vi "Teleop.vi"(10 "Match Info":T1={"Autonomous Elapsed Seconds"=0.0, "TeleOp Elapsed Seconds"=0.0, "Disabled Elapsed Seconds"=0.0, "Visited Autonomous"=FALSE, "Visited TeleOp"=FALSE, "Visited Disabled"=FALSE, "Autonomous Settings"={"Autonomous Style"=enum."Independent", "VI Refnum"=refnum}}, 11 "Call Context":T2) -> ()   [LabVIEW 2015]
doc: "This VI is called for each TeleOp packet received from the DS where the robot is not disabled. It is often used to read from the joysticks and update I/O or to update setpoints for timed control loops. It should complete and return within 20 milliseconds or it may miss DS packets."
uses:
  <vilib>/Rock Robotics/WPI/DriverStation/WPI_DriverStationDerivedRobotMode.ctl
  <vilib>/Rock Robotics/WPI/DriverStation/WPI_DriverStationMatch Info.ctl
  <vilib>/Rock Robotics/Network Tables/NT Read Boolean.vi
  <vilib>/Rock Robotics/Network Tables/NT Read Number.vi
  <vilib>/Rock Robotics/WPI/Utilities/WPI_GetSetVariantRefNum.vi
  <vilib>/Rock Robotics/Network Tables/NT Write Boolean Array.vi
  <vilib>/Rock Robotics/Network Tables/NT Write Numeric Array.vi
  <vilib>/Rock Robotics/Network Tables/NT Write Boolean.vi
  <vilib>/Rock Robotics/WPI/Solenoid/Deprecated/WPI_SolenoidSetBool.vi
  Sensors.vi
  Robot Global Data.vi
panel:
  in  "t":dbl=0.9
  in  "y":dbl=22500.0 format="%#_13g"
  out "Done":bool
  out "Drive Over":bool
  out "Start Climbing":bool
  out "Slow Turning":bool
  in  "Joystick Toning Factor":dbl=0.8 format="%#_13g"
  out "Release Climber Head":bool
  out "Release Climbing Solenoid":bool
  out "Break":bool
  out "Roller Open":bool
  out "Correct Wire":bool
  out "Alignment line shot":bool
  out "Low Goal":bool
  out "Lock Release":bool
  out "Auto Vision Tracking":bool
  out "High Goal shoot":bool
  out "High Goal prep":bool
  out "Intake Start":bool
  out "Sample Slider 0":dbl(slide) scale=0.0..5.0
  out "Sample Boolean 1":bool
  out "Sample Boolean 0":bool
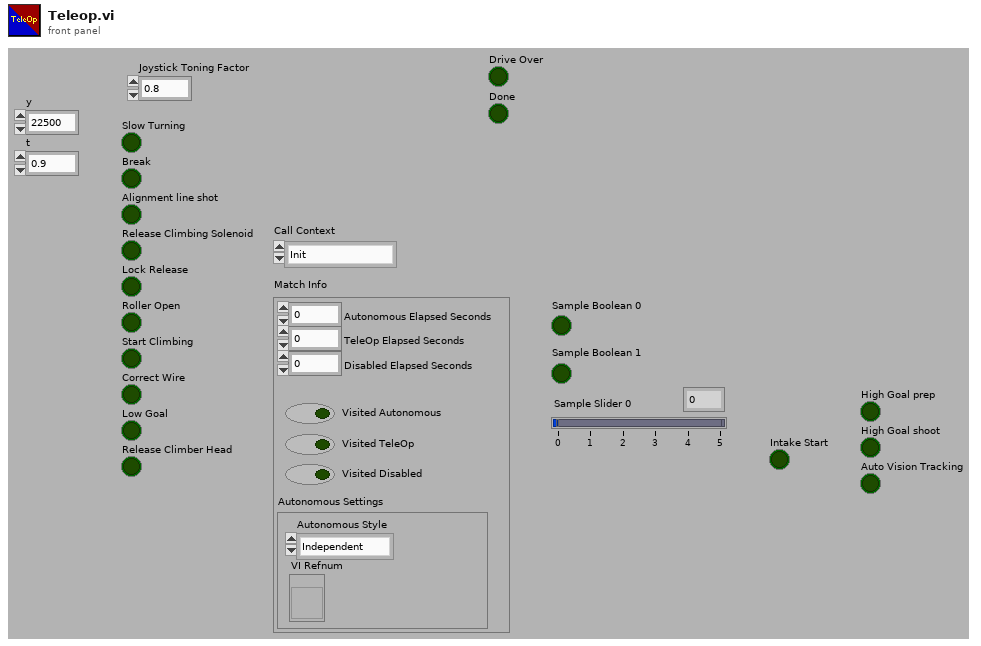
[diagram p1: front panel]
types:
  T1 = typedef "WPI_DriverStationMatch Info.ctl" = cluster{"Autonomous Elapsed Seconds":dbl, "TeleOp Elapsed Seconds":dbl, "Disabled Elapsed Seconds":dbl, "Visited Autonomous":bool, "Visited TeleOp":bool, "Visited Disabled":bool, "Autonomous Settings":cluster{"Autonomous Style":enum16{"Iterative", "Independent"}, "VI Refnum":refnum<vi>}}
  T2 = typedef "WPI_DriverStationDerivedRobotMode.ctl" = enum16{"Init", "Execute", "Stop"}
  T3 = typedef "WPI_JoystickDevRef.ctl" = cluster{"Device":T4}
  T4 = typedef "WPI_JoystickDeviceEnum.ctl" = enum16{"USB 0", "USB 1", "USB 2", "USB 3", "USB 4", "USB 5"}
  T5 = typedef "WPI_DigitalInputDevRef.ctl" = cluster{"DevStatus":errorcluster, "DIO Channel":T6}
  T6 = typedef "FPGA_DIOChannel.ctl" = enum8{"DIO 0", "DIO 1", "DIO 2", "DIO 3", "DIO 4", "DIO 5", "DIO 6", "DIO 7", "DIO 8", "DIO 9", "DIO MXP 0", "DIO MXP 1", "DIO MXP 2", "DIO MXP 3", "DIO MXP 4", "DIO MXP 5", "DIO MXP 6", "DIO MXP 7", "DIO MXP 8", "DIO MXP 9", "DIO MXP 10", "DIO MXP 11", "DIO MXP 12", "DIO MXP 13", "DIO MXP 14", "DIO MXP 15", "Invalid"}
  T7 = typedef "WPI_MotorControlDeviceRef.ctl" = cluster{"DeviceStatus":errorcluster, "Type":T8, "PWM":cluster{"PWM Channel":T9, "DeadBand":T10}, "CAN":cluster{"Device Number":u8, "Control Mode":T11, "Semaphore":T12, "Max Vout":dbl, "TalonSRX Control Mode":T13}, "Invert":bool}
  T8 = typedef "WPI_MotorControlType.ctl" = enum16{"PWM", "CAN", "CANTalonSRX"}
  T9 = typedef "FPGA_DIOPWMChannel.ctl" = enum8{"PWM 0", "PWM 1", "PWM 2", "PWM 3", "PWM 4", "PWM 5", "PWM 6", "PWM 7", "PWM 8", "PWM 9", "PWM MXP 0", "PWM MXP 1", "PWM MXP 2", "PWM MXP 3", "PWM MXP 4", "PWM MXP 5", "PWM MXP 6", "PWM MXP 7", "PWM MXP 8", "PWM MXP 9", "Invalid"}
  T10 = typedef "WPI_PWMDeadband.ctl" = cluster{"Name":string, "maxPositivePwm":i32, "minPositivePwm":i32, "centerPwm":i32, "maxNegativePwm":i32, "minNegativePwm":i32, "angularRange":u16}
  T11 = typedef "WPI_CANJaguar_ControlMode.ctl" = enum8{"Percent VBus", "Current", "Speed", "Position", "Voltage"}
  T12 = typedef "Semaphore RefNum" = refnum<k1>
  T13 = typedef "WPI_CANTalonSRX_APIControlMode.ctl" = enum8{"Percent VBus", "Speed", "Position", "Slave", "Unchanged / Invalid", "Voltage Compensation", "Current", "Motion Profile"}
  T14 = typedef "WPI_RobotDriveDevRef.ctl" = cluster{"DevStatus":errorcluster, "Motors[]":T7[], "Square Inputs":bool, "Max Output":dbl}
  T15 = typedef "WPI_SolenoidDevRef.ctl" = cluster{"DevStatus":errorcluster, "Pneumatics Control Module":u8, "Forward Solenoid Channel":T16, "Reverse Solenoid Channel":T16}
  T16 = typedef "WPI_SolenoidChannel.ctl" = enum8{"Solenoid 0", "Solenoid 1", "Solenoid 2", "Solenoid 3", "Solenoid 4", "Solenoid 5", "Solenoid 6", "Solenoid 7", "Invalid"}
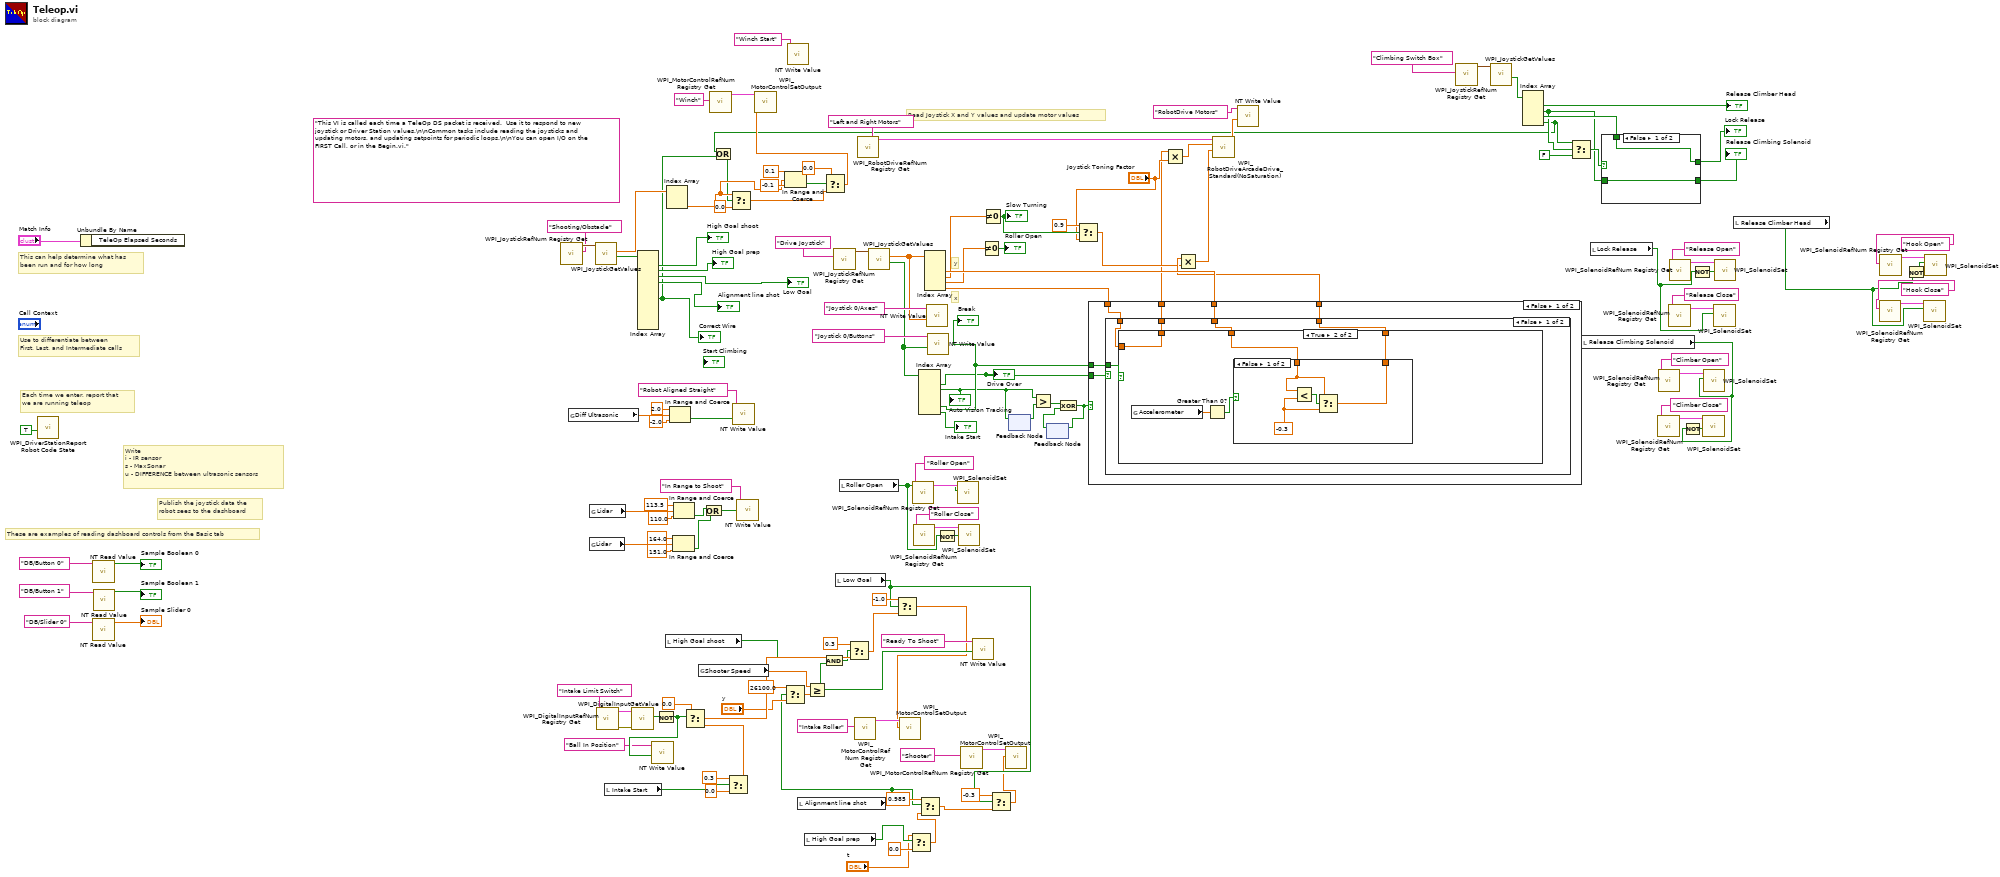
[diagram p0: block diagram]
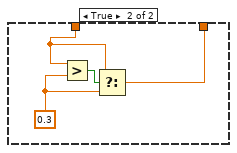
[diagram p3: hidden frame]
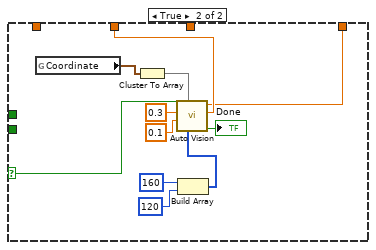
[diagram p5: hidden frame]
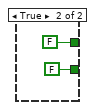
[diagram p6: hidden frame]
diagram:
  (unwired) "This VI is called each time a TeleOp DS packet is received.  Use it to respond to new joystick or Driver Station values.\n\nCommon tasks include reading the joysticks and updating motors, and updating setpoints for periodic loops.\n\nYou can open I/O on the FIRST Call, or in the Begin.vi."
  # "x"
  # "y"
  # "Read Joystick X and Y values and update motor values"
  # "Write\ni - IR sensor\ns - MaxSonar\nu - DIFFERENCE between ultrasonic sensors"
  # "These are examples of reading dashboard controls from the Basic tab"
  # "Publish the joystick data the\nrobot sees to the dashboard"
  # "Each time we enter, report that\nwe are running teleop"
  # "Use to differentiate between\nFirst, Last, and Intermediate calls"
  # "This can help determine what has\nbeen run and for how long"
  n1 = call <vilib>:"WPI_DriverStationReport Robot Code State.vi"("TeleOp"=TRUE ("Autonomous")) -> ()  [unwired: 10 in, 1 out]
  n2 = Unbundle By Name("Match Info") -> ()  [unwired: 1 out]
  n3 = call-poly <vilib>:"NT Read Value.vi"("Name"="DB/Button 0" ("refnum name")) -> ("Boolean"=→"Sample Boolean 0":bool)  [unwired: 9 in, 1 out]
  n4 = call-poly <vilib>:"NT Read Value.vi"("Name"="DB/Slider 0" ("refnum name")) -> ("Numeric"=→"Sample Slider 0":dbl)  [unwired: 9 in, 1 out]
  n5 = call-poly <vilib>:"NT Read Value.vi"("Name"="DB/Button 1" ("refnum name")) -> ("Boolean"=→"Sample Boolean 1":bool)  [unwired: 9 in, 1 out]
  n6 = call <vilib>:"WPI_JoystickRefNum Registry Get.vi"("refnum name"="Shooting/Obstacle") -> ("JoystickDevRef"=w122:T3)  [unwired: 1 in, 9 out]
  n7 = global read "Sensors.vi" "Diff Ultrasonic"() -> (w51:dbl)
  n8 = global read "Sensors.vi" "Lidar"() -> (w42:dbl)
  n9 = global read "Sensors.vi" "Lidar"() -> (w43:dbl)
  n10 = call <vilib>:"WPI_JoystickGetValues.vi"("JoystickDevRef"=w122) -> ("Buttons"=w120:bool[], "Axes"=w118:dbl[])  [unwired: 6 in, 3 out]
  n11 = call <vilib>:"WPI_DigitalInputRefNum Registry Get.vi"("refnum name"="Intake Limit Switch") -> ("error out"=w105:errorcluster, "DigitalInputDevRef"=w106:T5)  [unwired: 9 in]
  n12 = local read "Intake Start"() -> (w103:bool)
  n13 = call <vilib>:"WPI_DigitalInputGetValue.vi"("error in (no error)"=w105, "DigitalInputDevRef"=w106) -> ("Value"=w108:bool)  [unwired: 7 in, 2 out]
  n14 = Index Array(array=w120) -> (element #1=→"High Goal shoot":bool, element #2=→"High Goal prep":bool, element #3=→"Low Goal":bool, element #4=→"Alignment line shot":bool, element #7=w5:bool)  [unwired: 12 in, 7 out]
  "Correct Wire" <- w5
  n15 = Not(x=w108) -> (.not. x?=w58:bool)
  n16 = call-poly <vilib>:"NT Write Value.vi"("Boolean"=w58, "Name"="Ball In Position") -> ()  [unwired: 9 in, 1 out]
  n17 = local read "High Goal shoot"() -> (w95:bool)
  n18 = Index Array(array=w118) -> (element #2=w60:dbl)  [unwired: 2 in, 1 out]
  n19 = In Range and Coerce(upper limit=2.0, x=w51, lower limit=-2.0) -> (In Range?=w48:bool)  [unwired: 1 out]
  n20 = In Range and Coerce(upper limit=164.0, x=w42, lower limit=151.0) -> (In Range?=w38:bool)  [unwired: 1 out]
  n21 = In Range and Coerce(upper limit=113.5, x=w43, lower limit=110.0) -> (In Range?=w39:bool)  [unwired: 1 out]
  n22 = global read "Sensors.vi" "Shooter Speed"() -> (w1:dbl)
  n23 = Or(x=w39, y=w38) -> (x .or. y?=w37:bool)
  n24 = call <vilib>:"WPI_MotorControlRefNum Registry Get.vi"("refnum name"="Winch") -> ("MotorControlDevRef"=w80:T7)  [unwired: 9 in, 1 out]
  n25 = Select(t=0.3, s=w103, f=0.0) -> (s? t:f=w100:dbl)
  n26 = Select(t=0.0, s=w58, f=w100) -> (s? t:f=w99:dbl)
  n27 = call-poly <vilib>:"NT Write Value.vi"("Boolean"=w48, "Name"="Robot Aligned Straight") -> ()  [unwired: 9 in, 1 out]
  n28 = call-poly <vilib>:"NT Write Value.vi"("Boolean"=w37, "Name"="In Range to Shoot") -> ()  [unwired: 9 in, 1 out]
  n29 = In Range and Coerce(upper limit=0.1, x=w60, lower limit=-0.1) -> (In Range?=w76:bool)  [unwired: 1 out]
  n30 = call-poly <vilib>:"NT Write Value.vi"("Name"="Winch Start") -> ()  [unwired: 10 in, 1 out]
  n31 = local read "Alignment line shot"() -> (w29:bool)
  n32 = Select(t=26100.0, s=w29, f="y") -> (s? t:f=w30:dbl)
  n33 = local read "High Goal prep"() -> (w97:bool)
  n34 = Greater Or Equal?(x=w1, y=w30) -> (x >= y?=w55:bool)
  n35 = And(x=w95, y=w55) -> (x .and. y?=w94:bool)
  n36 = call <vilib>:"WPI_JoystickRefNum Registry Get.vi"("refnum name"="Drive Joystick") -> ("JoystickDevRef"=w128:T3)  [unwired: 1 in, 9 out]
  n37 = local read "Low Goal"() -> (w53:bool)
  n38 = local read "Roller Open"() -> (w109:bool)
  n39 = Select(t=0.3, s=w94, f=w99) -> (s? t:f=w111:dbl)
  n40 = call <vilib>:"WPI_MotorControlRefNum Registry Get.vi"("refnum name"="Intake Roller") -> ("MotorControlDevRef"=w132:T7)  [unwired: 9 in, 1 out]
  n41 = call <vilib>:"WPI_RobotDriveRefNum Registry Get.vi"("refnum name"="Left and Right Motors") -> ("RobotDriveDevRef"=w130:T14)  [unwired: 1 in, 9 out]
  n42 = call <vilib>:"WPI_JoystickGetValues.vi"("JoystickDevRef"=w128) -> ("Buttons"=w123:bool[], "Axes"=w119:dbl[])  [unwired: 6 in, 3 out]
  n43 = Select(t=-1.0, s=w53, f=w111) -> (s? t:f=w35:dbl)
  n44 = call <vilib>:"WPI_MotorControlSetOutput.vi"("Output"=w35, "MotorControlDevRef"=w132) -> ()  [unwired: 7 in, 3 out]
  n45 = Select(t="t", s=w97, f=0.0) -> (s? t:f=w28:dbl)
  n46 = call <vilib>:"WPI_SolenoidRefNum Registry Get.vi"("refnum name"="Roller Open") -> ("SolenoidDevRef"=w139:T15)  [unwired: 9 in, 1 out]
  n47 = call <vilib>:"WPI_SolenoidRefNum Registry Get.vi"("refnum name"="Roller Close") -> ("SolenoidDevRef"=w136:T15)  [unwired: 9 in, 1 out]
  n48 = Index Array(array=w123) -> (element #1=w36:bool, element #2=w12:bool, element #5=w92:bool, element #6=→"Intake Start":bool)  [unwired: 6 in, 2 out]
  "Auto Vision Tracking" <- w12
  "Break" <- w92
  "Drive Over" <- w36
  n49 = Select(t=0.985, s=w29, f=w28) -> (s? t:f=w32:dbl)
  n50 = Index Array(array=w119) -> (element #2=w93:dbl, element #3=w66:dbl, element #4=w69:dbl, element #5=w7:dbl)  [unwired: 5 in, 1 out]
  n51 = call-poly <vilib>:"NT Write Value.vi"("Numeric Array"=w119, "Name"="Joystick 0/Axes") -> ()  [unwired: 9 in, 1 out]
  n52 = call-poly <vilib>:"NT Write Value.vi"("Boolean Array"=w123, "Name"="Joystick 0/Buttons") -> ()  [unwired: 9 in, 1 out]
  n53 = Not(x=w109) -> (.not. x?=w135:bool)
  n54 = call-poly <vilib>:"WPI_SolenoidSet.vi"("Value"=w109, "SolenoidDevRef"=w139) -> ()  [unwired: 8 in, 2 out]
  n55 = call-poly <vilib>:"WPI_SolenoidSet.vi"("Value"=w135, "SolenoidDevRef"=w136) -> ()  [unwired: 8 in, 2 out]
  n56 = call <vilib>:"WPI_MotorControlRefNum Registry Get.vi"("refnum name"="Shooter") -> ("MotorControlDevRef"=w133:T7)  [unwired: 9 in, 1 out]
  n57 = call-poly <vilib>:"NT Write Value.vi"("Boolean"=w55, "Name"="Ready To Shoot") -> ()  [unwired: 9 in, 1 out]
  n58 = Not Equal To 0?(x=w69) -> (x != 0?=→"Roller Open":bool)
  n59 = Not Equal To 0?(x=w66) -> (x != 0?=w65:bool)
  "Slow Turning" <- w65
  n60 = Select(t=-0.3, s=w53, f=w32) -> (s? t:f=w34:dbl)
  n61 = call <vilib>:"WPI_MotorControlSetOutput.vi"("Output"=w34, "MotorControlDevRef"=w133) -> ()  [unwired: 7 in, 3 out]
  n62 = feedback-in #1(w12) -> ()
  n63 = feedback #1() -> (w13:bool)  [unwired: 1 in]
  n64 = Greater?(x=w12, y=w13) -> (0:w9:bool)
  n65 = feedback #2() -> (w10:bool)  [unwired: 1 in]
  n66 = Exclusive Or(1:w10, 2:w9) -> (0:w11:bool)
  n67 = feedback-in #2(w11) -> ()
  n68 = Select(t=0.9, s=w65, f="Joystick Toning Factor") -> (s? t:f=w62:dbl)
  n69 = case shown="False" w11 {
    selector: w11 -> [_ w182]
    tunnel: w93 -> [w154 _]
    tunnel: w92 -> [w153 _]
    tunnel: [w152 w177] -> w72
    tunnel: w36 -> [w151 _]
    tunnel: [w150 w178] -> w8
    tunnel: w7 -> [w149 _]
    frame False {
      n70 = case shown="False" w151 {
        tunnel: w154 -> [w159 w175]
        tunnel: w153 -> [w158 _]
        tunnel: [w157 w175] -> w152
        tunnel: [w156 w176] -> w150
        tunnel: w149 -> [w155 w176]
        frame False {
          n71 = case shown="True" w158 {
            tunnel: w159 -> [w161 w163]
            tunnel: [w161 w162] -> w157
            tunnel: [w160 w166] -> w156
            tunnel: w155 -> [w160 w166]
            frame False {
            }
            frame True {
              n72 = global read "Sensors.vi" "Accelerometer"() -> (w164:dbl)
              n73 = Greater Than 0?(x=w164) -> (x > 0?=w165:bool)
              n74 = case shown="False" w165 {
                tunnel: w163 -> [w168 w173]
                tunnel: [w167 w171] -> w162
                frame False {
                  w169 = -0.3
                  n75 = Less?(x=w168, y=w169) -> (x < y?=w170:bool)
                  n76 = Select(t=w168, s=w170, f=w169) -> (s? t:f=w167:dbl)
                }
                frame True {
                  w172 = 0.3
                  n77 = Greater?(x=w173, y=w172) -> (0:w174:bool)
                  n78 = Select(t=w173, s=w174, f=w172) -> (s? t:f=w171:dbl)
                }
              }
            }
          }
        }
        frame True {
        }
      }
    }
    frame True {
      n79 = global read "Robot Global Data.vi" "Coordinate"() -> (w185:cluster{"X":dbl, "Y":dbl})
      n80 = Cluster To Array(cluster=w185) -> (array=w183:dbl[])
      n81 = Build Array(160, 120) -> (w180:i32[])
      n82 = call "Auto Vision.vi"("Image Size"=w180, "Max Coordinate"=w183, "Rotational Velocity"=0.1, "Linear Velocity"=0.3, "Follow Colour ON"=w182) -> ("Done"=→"Done":bool, "Rotational Velocity_After"=w178:dbl, "Translational Velocity_After"=w177:dbl)  [unwired: 4 in]
    }
  }
  n83 = Multiply(x=w8, y="Joystick Toning Factor") -> (x*y=w73:dbl)
  n84 = Multiply(x=w72, y=w62) -> (x*y=w71:dbl)
  n85 = call <vilib>:"WPI_RobotDriveArcadeDrive_Standard(NoSaturation).vi"("Y axis value"=w71, "X axis value"=w73, "RobotDriveDevRef"=w130) -> ("Motor Values"=w125:dbl[])  [unwired: 1 in, 7 out]
  n86 = call-poly <vilib>:"NT Write Value.vi"("Numeric Array"=w125, "Name"="RobotDrive Motors") -> ()  [unwired: 9 in, 1 out]
  n87 = call <vilib>:"WPI_JoystickRefNum Registry Get.vi"("refnum name"="Climbing Switch Box") -> ("JoystickDevRef"=w26:T3)  [unwired: 1 in, 9 out]
  n88 = call <vilib>:"WPI_JoystickGetValues.vi"("JoystickDevRef"=w26) -> ("Buttons"=w24:bool[])  [unwired: 6 in, 4 out]
  n89 = Index Array(array=w24) -> (element #1=→"Release Climber Head":bool, element #2=w14:bool, element #3=w15:bool, element #4=w6:bool)  [unwired: 4 in]
  n90 = Or(x=w6, y=w5) -> (x .or. y?=w4:bool)
  n91 = Select(t=w60, s=w4, f=0.0) -> (s? t:f=w59:dbl)
  n92 = Select(t=0.0, s=w76, f=w59) -> (s? t:f=w74:dbl)
  n93 = call <vilib>:"WPI_MotorControlSetOutput.vi"("Output"=w74, "MotorControlDevRef"=w80) -> ()  [unwired: 7 in, 3 out]
  n94 = Select(t=w6, s=w14, f=FALSE) -> (s? t:f=w16:bool)
  n95 = local read "Release Climbing Solenoid"() -> (w23:bool)
  n96 = local read "Lock Release"() -> (w22:bool)
  n97 = case shown="False" w16 {
    tunnel: [w189 FALSE] -> w19
    tunnel: [w188 FALSE] -> w18
    tunnel: w15 -> [w189 _]
    tunnel: w14 -> [w188 _]
    frame False {
    }
    frame True {
    }
  }
  "Lock Release" <- w19
  "Release Climbing Solenoid" <- w18
  n98 = call <vilib>:"WPI_SolenoidRefNum Registry Get.vi"("refnum name"="Climber Close") -> ("SolenoidDevRef"=w113:T15)  [unwired: 9 in, 1 out]
  n99 = call <vilib>:"WPI_SolenoidRefNum Registry Get.vi"("refnum name"="Climber Open") -> ("SolenoidDevRef"=w116:T15)  [unwired: 9 in, 1 out]
  n100 = call <vilib>:"WPI_SolenoidRefNum Registry Get.vi"("refnum name"="Release Close") -> ("SolenoidDevRef"=w90:T15)  [unwired: 9 in, 1 out]
  n101 = call <vilib>:"WPI_SolenoidRefNum Registry Get.vi"("refnum name"="Release Open") -> ("SolenoidDevRef"=w87:T15)  [unwired: 9 in, 1 out]
  n102 = Not(x=w23) -> (.not. x?=w117:bool)
  n103 = Not(x=w22) -> (.not. x?=w81:bool)
  n104 = call-poly <vilib>:"WPI_SolenoidSet.vi"("Value"=w117, "SolenoidDevRef"=w113) -> ()  [unwired: 8 in, 2 out]
  n105 = call-poly <vilib>:"WPI_SolenoidSet.vi"("Value"=w23, "SolenoidDevRef"=w116) -> ()  [unwired: 8 in, 2 out]
  n106 = call-poly <vilib>:"WPI_SolenoidSet.vi"("Value"=w22, "SolenoidDevRef"=w90) -> ()  [unwired: 8 in, 2 out]
  n107 = call-poly <vilib>:"WPI_SolenoidSet.vi"("Value"=w81, "SolenoidDevRef"=w87) -> ()  [unwired: 8 in, 2 out]
  n108 = local read "Release Climber Head"() -> (w21:bool)
  n109 = call <vilib>:"WPI_SolenoidRefNum Registry Get.vi"("refnum name"="Hook Close") -> ("SolenoidDevRef"=w85:T15)  [unwired: 9 in, 1 out]
  n110 = call <vilib>:"WPI_SolenoidRefNum Registry Get.vi"("refnum name"="Hook Open") -> ("SolenoidDevRef"=w86:T15)  [unwired: 9 in, 1 out]
  n111 = Not(x=w21) -> (.not. x?=w82:bool)
  n112 = call-poly <vilib>:"WPI_SolenoidSet.vi"("Value"=w21, "SolenoidDevRef"=w85) -> ()  [unwired: 8 in, 2 out]
  n113 = call-poly <vilib>:"WPI_SolenoidSet.vi"("Value"=w82, "SolenoidDevRef"=w86) -> ()  [unwired: 8 in, 2 out]
